vi "open.vi"(8 "error in (no error)":errorcluster, 11 "MOXAIP in":refnum<class "MOXAIP.lvclass">) -> (0 "error out":errorcluster, 3 "MOXAIP out":refnum<class "MOXAIP.lvclass">)   [LabVIEW 2015, in "Serializer.lvlib" / "MOXAIP.lvclass"]
uses:
  MOXAIP.lvclass
  MOXAIP.lvclass/MOXAIP.ctl
  <vilib>/Utility/error.llb/Error Cluster From Error Code.vi
  <vilib>/ErrorRing/Error Ring.xnode
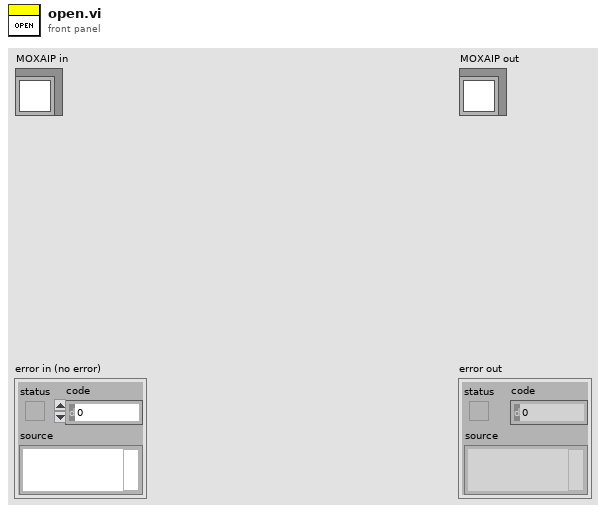
[diagram p1: front panel]
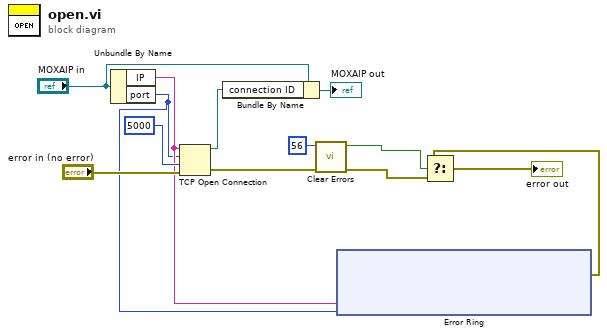
[diagram p0: block diagram]
diagram:
  n1 = Unbundle By Name("MOXAIP in") -> ("IP"=w2:string, "port"=w1:u16)
  n2 = TCP Open Connection(address=w2, remote port or service name=w1, timeout ms (60000)=5000, error in (no error)="error in (no error)") -> (connection ID=w10:refnum<k5>, error out=w8:errorcluster)  [unwired: 1 in]
  n3 = Bundle By Name(cluster="MOXAIP in", "connection ID"=w10) -> (→"MOXAIP out":refnum<class "MOXAIP.lvclass">)
  n4 = call <vilib>:"Clear Errors.vi"("error in (no error)"=w8, "specific error code to clear (0: all)"=56) -> ("error out"=w4:errorcluster, "specific error cleared?"=w6:bool)  [unwired: 4 in]
  n5 = xnode "Error Ring"("parameter 0"=w2, "parameter 1"=w1) -> ("error out"=w5:errorcluster)
  n6 = Select(t=w5, s=w6, f=w4) -> (s? t:f=→"error out":errorcluster)
